vi "Stoic_Mean_Calc.vi"(6 "Cycle Length":dbl, 8 "Multiple":dbl, 10 "Array In":dbl[](array[numeric])) -> (0 "Bin Array":dbl[](array[numeric]), 1 "Max":dbl format="%0.2f", 2 "Mean":dbl format="%0.2f", 3 "Min value":dbl, 4 "Temp Values":dbl[](array[numeric]), 5 "Max value":dbl, 7 "20% Bin Index":i32[](array[numeric]), 11 "20% value":dbl format="%#_13g")   [LabVIEW 2014]
uses:
  <vilib>/Analysis/baseanly.llb/Mean (DBL).vi
  <vilib>/Analysis/NI_AALBase.lvlib
panel:
  out "Max Array":dbl[](array[numeric])
  out "Mean Array":dbl[](array[numeric])
  out "Max Bin":dbl
  out "Min Bin":dbl
  # "Stoic Temperature Mean"
  # "Overall"
  # "Stoic"
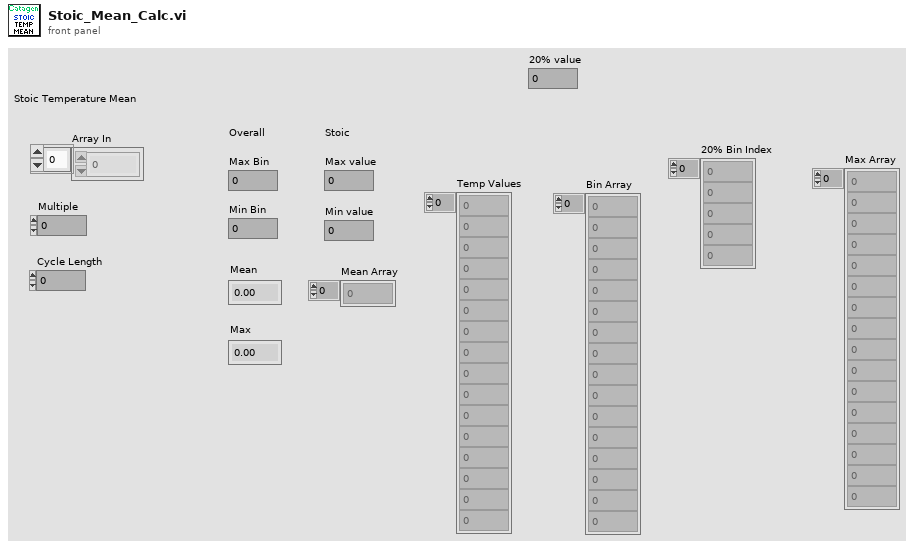
[diagram p1: front panel]
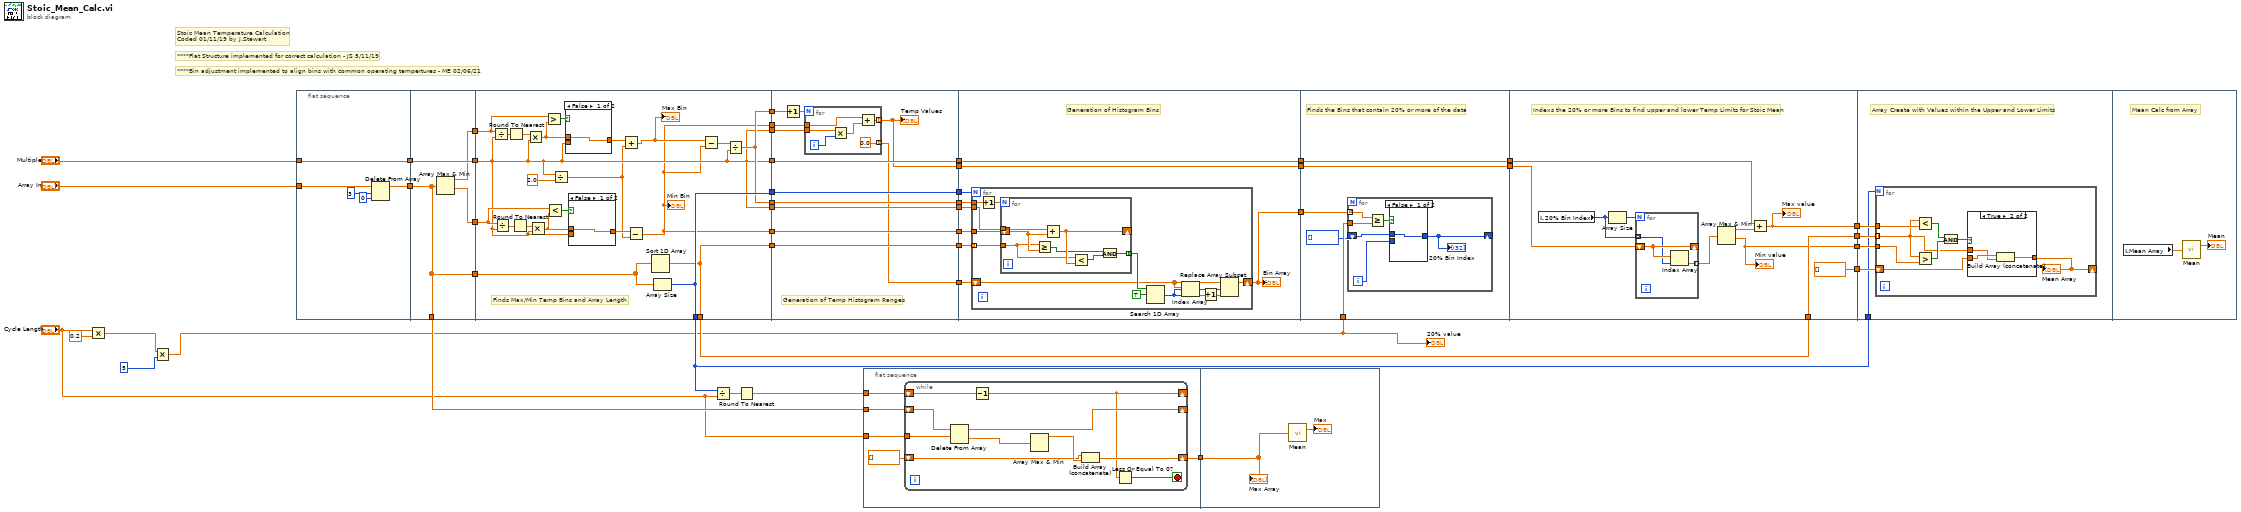
[diagram p0: block diagram]
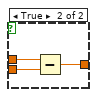
[diagram p2: hidden frame]
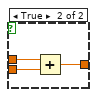
[diagram p3: hidden frame]
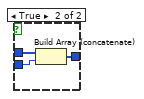
[diagram p4: hidden frame]
diagram:
  # "****Bin adjustment implemented to align bins with common operating tempertures - ME 02/06/21"
  # "****Flat Structure implemented for correct calculation - JS 5/11/19"
  # "Stoic Mean Temperature Calculation\nCoded 01/11/19 by J.Stewart"
  n1 = Multiply(x="Cycle Length", y=0.2) -> (x*y=w2:dbl)
  n2 = Multiply(x=w2, y=5) -> (x*y=w1:dbl)
  "20% value" <- w1
  n3 = flat-sequence {
    tunnel: "Multiple" -> [w50]
    tunnel: [w50] -> w12
    tunnel: [w47] -> w11
    tunnel: "Array In" -> [w46]
    tunnel: [w54] -> w16
    tunnel: [w51] -> w15
    tunnel: [w53] -> w14
    tunnel: [w52] -> w13
    tunnel: w12 -> [w54]
    tunnel: w11 -> [w51]
    tunnel: [w51] -> w7
    tunnel: [w74] -> w26
    tunnel: [w56] -> w25
    tunnel: [w60] -> w24
    tunnel: [w73] -> w23
    tunnel: [w75] -> w22
    tunnel: [w60] -> w21
    tunnel: [w73] -> w20
    tunnel: [w56] -> w19
    tunnel: [w75] -> w9
    tunnel: [w74] -> w18
    tunnel: [w60] -> w17
    tunnel: w16 -> [w60]
    tunnel: w15 -> [w76]
    tunnel: w14 -> [w67]
    tunnel: w13 -> [w62]
    tunnel: [w89] -> w39
    tunnel: [w96] -> w38
    tunnel: [w95] -> w37
    tunnel: [w94] -> w36
    tunnel: [w93] -> w35
    tunnel: [w92] -> w34
    tunnel: [w85] -> w32
    tunnel: [w91] -> w29
    tunnel: w26 -> [w96]
    tunnel: w25 -> [w95]
    tunnel: w24 -> [w94]
    tunnel: w23 -> [w93]
    tunnel: w22 -> [w92]
    tunnel: w21 -> [w91]
    tunnel: w20 -> [w88]
    tunnel: w19 -> [w86]
    tunnel: w17 -> [w87]
    tunnel: [w111] -> w40
    tunnel: w39 -> [w110]
    tunnel: w38 -> [w109]
    tunnel: w37 -> [w108]
    tunnel: w36 -> [w107]
    tunnel: w35 -> [w106]
    tunnel: w34 -> [w105]
    tunnel: w32 -> [w104]
    tunnel: [w104] -> w31
    tunnel: w29 -> [w103]
    tunnel: [w103] -> w28
    tunnel: w1 -> [w134]
    tunnel: w40 -> [w135]
    tunnel: [w132] -> w33
    tunnel: w31 -> [w132]
    tunnel: [w131] -> w30
    tunnel: w28 -> [w131]
    tunnel: w18 -> [w155]
    tunnel: [w150] -> w44
    tunnel: [dbl[] [] ("Array 3")] -> w43
    tunnel: [w155] -> w42
    tunnel: [w149] -> w41
    tunnel: w33 -> [w147]
    tunnel: w30 -> [w146]
    tunnel: w44 -> [w162]
    tunnel: w43 -> [w161]
    tunnel: w42 -> [w160]
    tunnel: w41 -> [w163]
    tunnel: w9 -> [w159]
    frame #0 {
      n4 = Delete From Array(array=w46, length=3, index=0) -> (array with subset deleted=w47:dbl[])  [unwired: 1 out]
    }
    frame #1 {
      n5 = Array Max & Min(array=w51) -> (max value=w53:dbl, min value=w52:dbl)  [unwired: 2 out]
    }
    frame #2 {
      # "Finds Max/Min Temp Bins and Array Length"
      n6 = Divide(x=w67, y=w60) -> (x/y=w68:dbl)
      n7 = Divide(x=w62, y=w60) -> (x/y=w63:dbl)
      n8 = Round To Nearest(number=w68) -> (nearest integer value=w69:dbl)
      n9 = Round To Nearest(number=w63) -> (nearest integer value=w64:dbl)
      n10 = Multiply(x=w69, y=w60) -> (x*y=w70:dbl)
      n11 = Multiply(x=w64, y=w60) -> (x*y=w65:dbl)
      n12 = Greater?(x=w67, y=w70) -> (0:w71:bool)
      n13 = Less?(x=w62, y=w65) -> (x < y?=w66:bool)
      n14 = Divide(x=w60, y=2.0) -> (x/y=w55:dbl)
      n15 = case shown="False" w71 {
        tunnel: w70 -> [w81 w84]
        tunnel: w60 -> [_ w83]
        tunnel: [w81 w82] -> w59
        frame False {
        }
        frame True {
          n16 = Add(x=w84, y=w83) -> (x+y=w82:dbl)
        }
      }
      n17 = case shown="False" w66 {
        tunnel: w65 -> [w77 w80]
        tunnel: w60 -> [_ w79]
        tunnel: [w77 w78] -> w57
        frame False {
        }
        frame True {
          n18 = Subtract(x=w80, y=w79) -> (x-y=w78:dbl)
        }
      }
      n19 = Add(x=w59, y=w55) -> (x+y=w58:dbl)
      "Max Bin" <- w58
      n20 = Subtract(x=w57, y=w55) -> (x-y=w56:dbl)
      "Min Bin" <- w56
      n21 = Sort 1D Array(array=w76) -> (sorted array=w74:dbl[])
      n22 = Array Size(array=w76) -> (size(s)=w75:i32)
      n23 = Subtract(x=w58, y=w56) -> (x-y=w72:dbl)
      n24 = Divide(x=w72, y=w60) -> (x/y=w73:dbl)
    }
    frame #3 {
      # "Generation of Temp Histogram Ranges"
      n25 = Increment(x=w88) -> (x+1=w90:dbl)
      n26 = for {
        N: w90 -> [_]
        tunnel: w87 -> [w102]
        tunnel: w86 -> [w101]
        tunnel: [w99] -> w85 mode=indexing
        tunnel: [0.0 ("x+y")] -> w89 mode=indexing
        i -> [w98]
        n27 = Multiply(x=w102, y=w98) -> (x*y=w100:dbl)
        n28 = Add(x=w101, y=w100) -> (x+y=w99:dbl)
      }
      "Temp Values" <- w85
    }
    frame #4 {
      # "Generation of Histogram Bins"
      n29 = for {
        N: w105 -> [_]
        tunnel: w107 -> [w122]
        tunnel: w109 -> [w123] mode=indexing
        tunnel: w106 -> [w112]
        tunnel: w108 -> [w121]
        shift-right: [w120] -> w111
        shift-left: w110 -> [w116]
        n30 = Increment(x=w112) -> (x+1=w113:dbl)
        n31 = for {
          N: w113 -> [_]
          tunnel: w123 -> [w126]
          tunnel: w122 -> [w124]
          shift-right: [w129] -> _
          shift-left: w121 -> [w130]
          tunnel: [w125] -> w119 mode=indexing
          n32 = Greater Or Equal?(x=w126, y=w130) -> (x >= y?=w127:bool)
          n33 = Add(x=w124, y=w130) -> (x+y=w129:dbl)
          n34 = Less?(x=w126, y=w129) -> (x < y?=w128:bool)
          n35 = And(x=w127, y=w128) -> (x .and. y?=w125:bool)
        }
        n36 = Search 1D Array(1D array=w119, element=TRUE) -> (index of element=w117:i32)  [unwired: 1 in]
        n37 = Index Array(array=w116, index=w117) -> (element=w115:dbl)
        n38 = Increment(x=w115) -> (x+1=w114:dbl)
        n39 = Replace Array Subset(array=w116, new element=w114, index=w117) -> (w120:dbl[])
      }
      "Bin Array" <- w111
    }
    frame #5 {
      # "Finds the Bins that contain 20% or more of the data"
      n40 = for {
        tunnel: w135 -> [w141] mode=indexing
        shift-right: [w138] -> _
        shift-left: i32[] [] -> [w137]
        tunnel: w134 -> [w136]
        i -> [w139]
        n41 = Greater Or Equal?(x=w141, y=w136) -> (x >= y?=w140:bool)
        n42 = case shown="False" w140 {
          tunnel: w139 -> [_ w145]
          tunnel: [w142 w144] -> w138
          tunnel: w137 -> [w142 w143]
          frame False {
          }
          frame True {
            n43 = Build Array (concatenate)(w143, w145) -> (w144:i32[])
          }
        }
        "20% Bin Index" <- w138
      }
    }
    frame #6 {
      # "Indexs the 20% or more Bins to find upper and lower Temp Limits for Stoic Mean"
      n44 = local read "20% Bin Index"() -> (w148:i32[])
      n45 = Array Size(array=w148) -> (size(s)=w151:i32)
      n46 = for {
        N: w151 -> [_]
        tunnel: w148 -> [w157] mode=indexing
        shift-right: [w158] -> _
        shift-left: w147 -> [w158]
        tunnel: [w156] -> w152 mode=indexing
        n47 = Index Array(array=w158, index=w157) -> (element=w156:dbl)
      }
      n48 = Array Max & Min(array=w152) -> (max value=w153:dbl, min value=w149:dbl)  [unwired: 2 out]
      "Min value" <- w149
      n49 = Add(x=w146, y=w153) -> (x+y=w150:dbl)
      "Max value" <- w150
    }
    frame #7 {
      # "Array Create with Values within the Upper and Lower Limits"
      n50 = for {
        N: w159 -> [_]
        tunnel: w163 -> [w171]
        tunnel: w162 -> [w170]
        shift-right: [w164] -> _
        shift-left: w161 -> [w166]
        tunnel: w160 -> [w165] mode=indexing
        n51 = Less?(x=w165, y=w170) -> (x < y?=w169:bool)
        n52 = Greater?(x=w165, y=w171) -> (0:w168:bool)
        n53 = And(x=w169, y=w168) -> (x .and. y?=w167:bool)
        n54 = case shown="True" w167 {
          tunnel: w166 -> [w172 w175]
          tunnel: [w172 w174] -> w164
          tunnel: w165 -> [_ w173]
          frame False {
          }
          frame True {
            n55 = Build Array (concatenate)(w175, w173) -> (w174:dbl[])
          }
        }
        "Mean Array" <- w164
      }
    }
    frame #8 {
      # "Mean Calc from Array"
      n56 = local read "Mean Array"() -> (w177:dbl[])
      n57 = call-poly <vilib>:"Mean.vi"("X"=w177) -> ("mean"=→"Mean":dbl)  [unwired: 1 out]
    }
  }
  n58 = Divide(x=w9, y="Cycle Length") -> (x/y=w8:dbl)
  n59 = Round To Nearest(number=w8) -> (nearest integer value=w6:dbl)
  n60 = flat-sequence {
    tunnel: w7 -> [w182]
    tunnel: w6 -> [w181]
    tunnel: "Cycle Length" -> [w180]
    tunnel: [w178] -> w4
    tunnel: w4 -> [w193]
    frame #0 {
      n61 = while {
        shift-right: [w190] -> _
        shift-left: w182 -> [w192]
        tunnel: w180 -> [w191]
        shift-right: [w188] -> w178
        shift-left: dbl[] [] -> [w186]
        shift-right: [w183] -> _
        shift-left: w181 -> [w184]
        stop <- w185 stop-if-true
        n62 = Delete From Array(array=w192, length=w191) -> (deleted portion=w189:dbl[], array with subset deleted=w190:dbl[])  [unwired: 1 in]
        n63 = Decrement(x=w184) -> (x-1=w183:dbl)
        n64 = Array Max & Min(array=w189) -> (max value=w187:dbl)  [unwired: 3 out]
        n65 = Build Array (concatenate)(w186, w187) -> (w188:dbl[])
        n66 = Less Or Equal To 0?(x=w183) -> (x <= 0?=w185:bool)
      }
    }
    frame #1 {
      n67 = call-poly <vilib>:"Mean.vi"("X"=w193) -> ("mean"=→"Max":dbl)  [unwired: 1 out]
      "Max Array" <- w193
    }
  }
